vi "Controller Open Synchronization Objects.vi"(8 "error in (no error)":errorcluster, 11 "FOFB Configuration":T5={"FOFB Parameters"={"Network"={"FOFB Controller IP"="", "LNLS Control Network IP"="", "LNLS Control Network Power Supplies TCP Port"=0, "LNLS Control Network FOFB Configuration TCP Port"=0, "Data Server TCP Port"=0, "Monitoring Data TCP Port"=0, "Configuration GUI TCP Port"=0, "TCP Listening Timeout"=0}, "Fast Acquisition"={"Acquisition Period"=0, "Data Buffer Size"=0, "Monitoring Period"=0}, "Response Matrix Measurement"={"Step Amplitude"=0.0, "Time Between Steps"=0, "Step Duration"=0, "Number of Averages"=0}, "Correction Algorithm"={"Correction Period"=0, "Reference Orbit Path"=path "", "Response Matrix Path"=path "", "Correction Matrix Path"=path "", "Horizontal Correction Factor"=0.0, "Vertical Correction Factor"=0.0, "Beam Current FOFB Threshold"=0.0, "Decouple H-V"=FALSE, "Use Additional BPM LPF"=FALSE, "BPM LPF Cutoff"=0.0}, "Acquisition Network"=[], "Actuation Network"=[]}, "Number of Acquisition Chassis"=0, "Number of Actuation Chassis"=0, "Number of BPM Readings"=0, "BPM Reading Names"=[], "Selected BPM Readings"=[0, 1, 2, 3, 4, 5, 6, 7, 8, 9, 10, 11, 12, 13, 14, 15, 16, 17, 18, 19, 20, 21, 22, 23, 24, 25, 26, 27, 28, 29, 30, 31, 32, 33, 34, 35, 36, 37, 38, 39, 40, 41, 42, 43, 44, 45, 46, 47, 48, 49], "Number of Correctors"=0, "Corrector Names"=[], "Selected Correctors"=[0, 1, 2, 3, 4, 5, 6, 7, 8, 9, 10, 11, 12, 13, 14, 15, 16, 17, 18, 19, 20, 21, 22, 23, 24, 25, 26, 27, 28, 29, 30, 31, 32, 33, 34, 35, 36, 37, 38, 39, 40, 41, 42, 43, 44, 45, 46, 47, 48, 49], "Reference Orbit"=[], "Response Matrix"=[], "Correction Matrix"=[], "Acquisition Chassis Names"=[], "Actuation Chassis Names"=[], "Acquisition Variables"=[], "Actuation Variables"=[], "PS Matrix Mapping"=[], "Inverse PS Matrix Mapping"=[], "Response Matrix Beam Energy (MeV)"=0.0, "PID Parameters"=[], "BPM Planes"=[], "Corrector Planes"=[], "RMM Step Factor"=[]}) -> (0 "error out":errorcluster, 3 "Sync Objects":T1)   [LabVIEW 2011, in "Controller VIs.lvlib"]
uses:
  Controller VIs.lvlib
  Types Definitions/Type FOFB Configuration.ctl
  Types Definitions/Type FOFB Parameters.ctl
  Types Definitions/Type Network Configuration.ctl
  Types Definitions/Type FA Configuration.ctl
  Types Definitions/Type Response Matrix Measurement Configuration.ctl
  Types Definitions/Type Correction Algorithm Configuration.ctl
  Types Definitions/Type Acquisition Network Configuration.ctl
  Types Definitions/Type Actuation Network Configuration.ctl
  Types Definitions/Type PID Parameters.ctl
  Types Definitions/Type Synchronization Objects.ctl
  Types Definitions/Type Blocking Synchronization Objects.ctl
  Types Definitions/Type FA Request Parameters.ctl
  Types Definitions/Type BPM and PS select cluster.ctl
  Types Definitions/Type FA File Parameters.ctl
  Types Definitions/Type Monitoring Data.ctl
  Types Definitions/Type Diagnostics Data.ctl
  Types Definitions/Type CPU Loads Array.ctl
  Types Definitions/Type CPU Loads.ctl
  Types Definitions/Type Non-blocking Synchronization Objects.ctl
  Types Definitions/Type FOFB Variables.ctl
  Types Definitions/Type Actuation State.ctl
  Type Definitions.lvlib
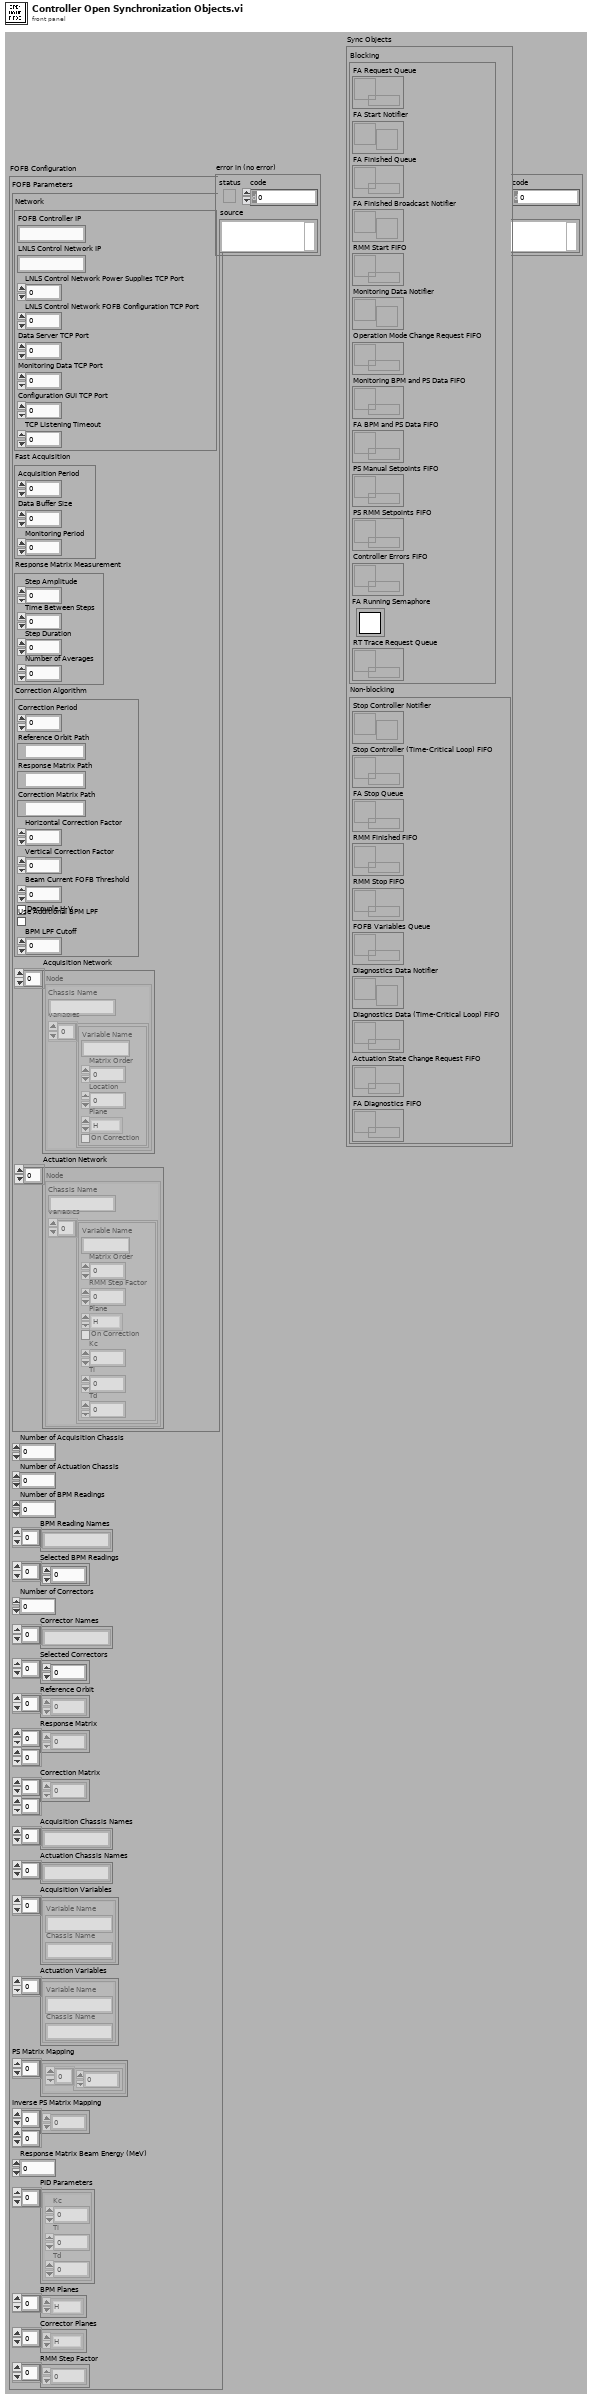
[diagram p1: front panel]
types:
  T1 = typedef "Type Definitions.lvlib/Type Synchronization Objects.ctl" = cluster{"Blocking":T2, "Non-blocking":T4}
  T2 = typedef "Type Definitions.lvlib/Type Blocking Synchronization Objects.ctl" = cluster{"FA Request Queue":refnum<queue>, "FA Start Notifier":refnum<notifier>, "FA Finished Queue":refnum<queue>, "FA Finished Broadcast Notifier":refnum<notifier>, "RMM Start FIFO":refnum<k33>, "Monitoring Data Notifier":refnum<notifier>, "Operation Mode Change Request FIFO":refnum<k33>, "Monitoring BPM and PS Data FIFO":refnum<k33>, "FA BPM and PS Data FIFO":refnum<k33>, "PS Manual Setpoints FIFO":refnum<k33>, "PS RMM Setpoints FIFO":refnum<k33>, "Controller Errors FIFO":refnum<k33>, "FA Running Semaphore":T3, "RT Trace Request Queue":refnum<queue>}
  T3 = typedef "Semaphore RefNum" = refnum<k1>
  T4 = typedef "Type Definitions.lvlib/Type Non-blocking Synchronization Objects.ctl" = cluster{"Stop Controller Notifier":refnum<notifier>, "Stop Controller (Time-Critical Loop) FIFO":refnum<k33>, "FA Stop Queue":refnum<queue>, "RMM Finished FIFO":refnum<k33>, "RMM Stop FIFO":refnum<k33>, "FOFB Variables Queue":refnum<queue>, "Diagnostics Data Notifier":refnum<notifier>, "Diagnostics Data (Time-Critical Loop) FIFO":refnum<k33>, "Actuation State Change Request FIFO":refnum<k33>, "FA Diagnostics FIFO":refnum<k33>}
  T5 = typedef "Type Definitions.lvlib/Type FOFB Configuration.ctl" = cluster{"FOFB Parameters":T6, "Number of Acquisition Chassis":i32, "Number of Actuation Chassis":i32, "Number of BPM Readings":i32, "BPM Reading Names":string[], "Selected BPM Readings":u32[], "Number of Correctors":i32, "Corrector Names":string[], "Selected Correctors":u32[], "Reference Orbit":dbl[], "Response Matrix":dbl[][], "Correction Matrix":dbl[][], "Acquisition Chassis Names":string[], "Actuation Chassis Names":string[], "Acquisition Variables":cluster{"Variable Name":string, "Chassis Name":string}[], "Actuation Variables":cluster{"Variable Name":string, "Chassis Name":string}[], "PS Matrix Mapping":cluster{u32[]}[], "Inverse PS Matrix Mapping":u32[][], "Response Matrix Beam Energy (MeV)":dbl, "PID Parameters":T13[], "BPM Planes":enum8{"H", "V"}[], "Corrector Planes":enum8{"H", "V"}[], "RMM Step Factor":dbl[]}
  T6 = typedef "Type Definitions.lvlib/Type FOFB Parameters.ctl" = cluster{"Network":T7, "Fast Acquisition":T8, "Response Matrix Measurement":T9, "Correction Algorithm":T10, "Acquisition Network":T11, "Actuation Network":T12}
  T7 = typedef "Type Definitions.lvlib/Type Network Configuration.ctl" = cluster{"FOFB Controller IP":string, "LNLS Control Network IP":string, "LNLS Control Network Power Supplies TCP Port":u16, "LNLS Control Network FOFB Configuration TCP Port":u16, "Data Server TCP Port":u16, "Monitoring Data TCP Port":u16, "Configuration GUI TCP Port":u16, "TCP Listening Timeout":i32}
  T8 = typedef "Type Definitions.lvlib/Type FA Configuration.ctl" = cluster{"Acquisition Period":u32, "Data Buffer Size":u32, "Monitoring Period":u32}
  T9 = typedef "Type Definitions.lvlib/Type Response Matrix Measurement Configuration.ctl" = cluster{"Step Amplitude":dbl, "Time Between Steps":u32, "Step Duration":u32, "Number of Averages":u32}
  T10 = typedef "Type Definitions.lvlib/Type Correction Algorithm Configuration.ctl" = cluster{"Correction Period":u32, "Reference Orbit Path":path, "Response Matrix Path":path, "Correction Matrix Path":path, "Horizontal Correction Factor":dbl, "Vertical Correction Factor":dbl, "Beam Current FOFB Threshold":dbl, "Decouple H-V":bool, "Use Additional BPM LPF":bool, "BPM LPF Cutoff":dbl}
  T11 = typedef "Type Definitions.lvlib/Type Acquisition Network Configuration.ctl" = cluster{"Chassis Name":string, "Variables":cluster{"Variable Name":string, "Matrix Order":u32, "Location":dbl, "Plane":enum8{"H", "V"}, "On Correction":bool}[]}[]
  T12 = typedef "Type Definitions.lvlib/Type Actuation Network Configuration.ctl" = cluster{"Chassis Name":string, "Variables":cluster{"Variable Name":string, "Matrix Order":u32, "RMM Step Factor":dbl, "Plane":enum8{"H", "V"}, "On Correction":bool, "Kc":dbl, "Ti":dbl, "Td":dbl}[]}[]
  T13 = typedef "Type Definitions.lvlib/Type PID Parameters.ctl" = cluster{"Kc":fxp<+/-,16,8>, "Ti":fxp<+/-,16,8>, "Td":fxp<+/-,16,8>}
  T14 = typedef "Type Definitions.lvlib/Type FOFB Variables.ctl" = cluster{"Correction Period":u32, "Reference Orbit":dbl[], "Response Matrix":dbl[][], "Correction Matrix":dbl[][], "Decouple H-V":bool, "Horizontal Correction Factor":dbl, "Vertical Correction Factor":dbl, "Selected BPM Readings":u32[], "Selected Correctors":u32[], "BPM Planes":enum8{"H", "V"}[], "Corrector Planes":enum8{"H", "V"}[], "Beam Current FOFB Threshold":dbl, "Response Matrix Beam Energy (MeV)":dbl}
  T15 = typedef "Type Definitions.lvlib/Type FA File Parameters.ctl" = cluster{"FA Parameters":T16, "File Reference":refnum<file>}
  T16 = typedef "Type Definitions.lvlib/Type FA Request Parameters.ctl" = cluster{"Number of Samples":u32, "BPM and PS Selection":T17, "Filename":string}
  T17 = typedef "Type Definitions.lvlib/Type BPM and PS select cluster.ctl" = cluster{"BPM index array":u32[], "PS index array ":u32[]}
  T18 = cluster{"read mode":enum16{"polling", "blocking"}, "write mode":enum16{"polling", "blocking"}}
  T19 = typedef "Type Definitions.lvlib/Type Diagnostics Data.ctl" = cluster{"Time-Critical Loop Missed Iterations":u32, "Time-Critical Loop Execution Time (usec)":u32, "FA Buffer Usage":u32, "Available Memory (bytes)":u32, "CPU Loads Array":T20}
  T20 = typedef "Type Definitions.lvlib/Type CPU Loads Array.ctl" = T21[]
  T21 = typedef "Type Definitions.lvlib/Type CPU Loads.ctl" = cluster{"Total (%)":dbl, "Time Critical (%)":dbl, "Timed Structures (%)":dbl, "High (%)":dbl, "Above Normal (%)":dbl, "Normal (%)":dbl, "Background (%)":dbl, "Idle (%)":dbl, "ISR (%)":dbl}
  T22 = typedef "Type Definitions.lvlib/Type Monitoring Data.ctl" = cluster{"Timestamp":timestamp, "BPM Readings":dbl[], "PS Readings":dbl[], "PS FOFB Setpoints":dbl[], "PS Status per Rack":u8[], "PS ON-OFF per Rack":u8[], "Operation Mode":enum16{"Idle Mode", "Error Mode", "Manual Mode", "FOFB Mode", "RMM Mode"}, "Diagnostics Data":T19, "Controller Status Table":i32[]}
  T23 = enum16{"Idle Mode", "Error Mode", "Manual Mode", "FOFB Mode", "RMM Mode"}
  T24 = typedef "Type Definitions.lvlib/Type Actuation State.ctl" = enum16{"Only reading", "Manual", "FOFB Initialization", "FOFB", "FOFB Stopping", "RMM Initialization", "RMM", "RMM Stopping"}
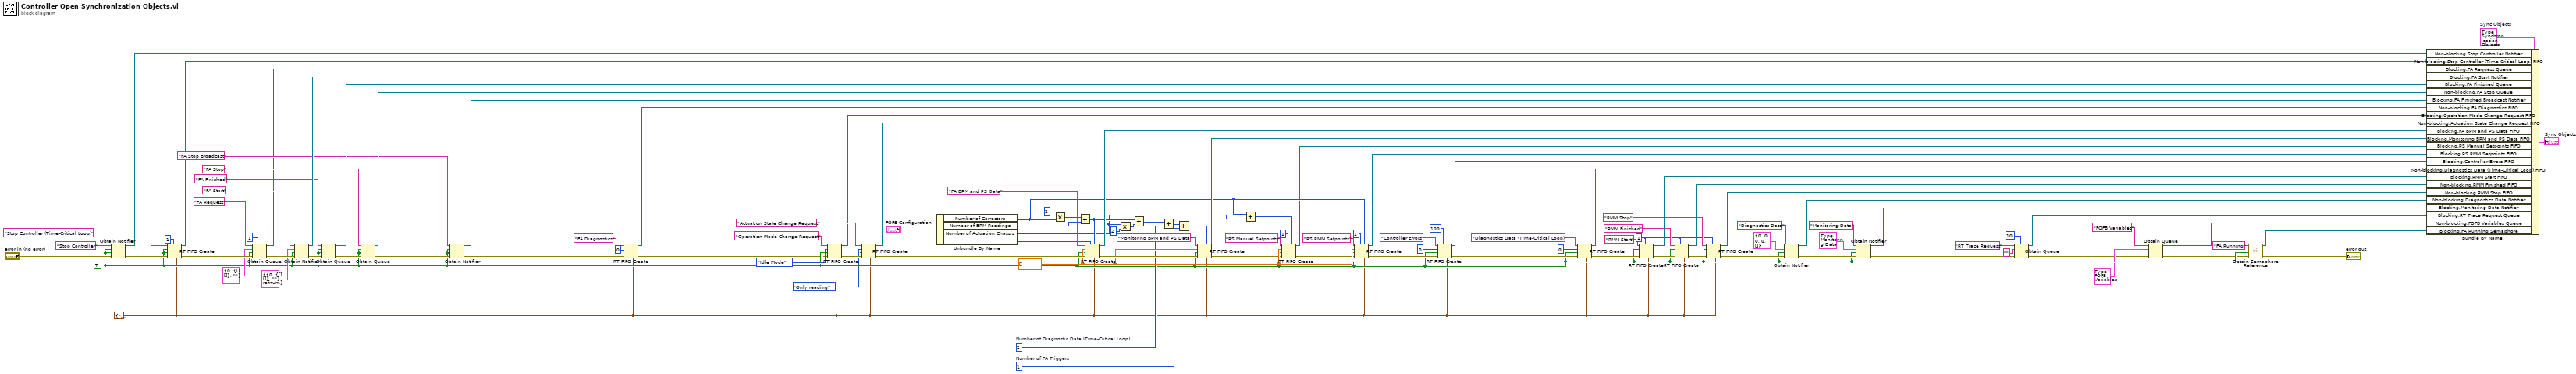
[diagram p0: block diagram]
diagram:
  w7 = 1  # Number of FA Triggers
  w30 = 2  # Number of Diagnostic Data (Time-Critical Loop)
  w11 = T18 {"read mode"=enum."blocking", "write mode"=enum."blocking"} ("r/w modes (polling,polling)")
  w58 = u32 1 ("size (10)")
  w104 = T1 {"Blocking"={"FA Request Queue"=refnum, "FA Start Notifier"=refnum, "FA Finished Queue"=refnum, "FA Finished Broadcast Notifier"=refnum, "RMM Start FIFO"=refnum, "Monitoring Data Notifier"=refnum, "Operation Mode Change Request FIFO"=refnum, "Monitoring BPM and PS Data FIFO"=refnum, "FA BPM and PS Data FIFO"=refnum, "PS Manual Setpoints FIFO"=refnum, "PS RMM Setpoints FIFO"=refnum, "Controller Errors FIFO"=refnum, "FA Running Semaphore"=refnum, "RT Trace Request Queue"=refnum}, "Non-blocking"={"Stop Controller Notifier"=refnum, "Stop Controller (Time-Critical Loop) FIFO"=refnum, "FA Stop Queue"=refnum, "RMM Finished FIFO"=refnum, "RMM Stop FIFO"=refnum, "FOFB Variables Queue"=refnum, "Diagnostics Data Notifier"=refnum, "Diagnostics Data (Time-Critical Loop) FIFO"=refnum, "Actuation State Change Request FIFO"=refnum, "FA Diagnostics FIFO"=refnum}}  # Sync Objects
  w22 = TRUE
  w46 = dbl[] [] ("BPM Readings")
  n1 = Obtain Notifier(name (unnamed)="Stop Controller", notification data type=w22, create if not found? (T)=w22, error in (no error)="error in (no error)") -> (notifier out=w105:refnum<notifier>, error out=w56:errorcluster)  [unwired: 1 out]
  n2 = RT FIFO Create(0:"Stop Controller (Time-Critical Loop)" ("name (unnamed)"), 1:w22, 2:w22, 3:w56, 4:u32 1 ("size (10)"), 7:w11) -> (8:w52:refnum<k33>, 11:w55:errorcluster)  [unwired: 2 in, 1 out]
  n3 = Obtain Queue(max queue size (-1, unlimited)=1, name (unnamed)="FA Request", element data type=T16 {"Number of Samples"=0, "BPM and PS Selection"={"BPM index array"=[], "PS index array "=[]}, "Filename"=""} ("Acquisition Period"), create if not found? (T)=w22, error in (no error)=w55) -> (queue out=w16:refnum<queue>, error out=w97:errorcluster)  [unwired: 1 out]
  n4 = Obtain Notifier(name (unnamed)="FA Start", notification data type=T15 {"FA Parameters"={"Number of Samples"=0, "BPM and PS Selection"={"BPM index array"=[], "PS index array "=[]}, "Filename"=""}, "File Reference"=refnum} ("File Parameters"), create if not found? (T)=w22, error in (no error)=w97) -> (notifier out=w106:refnum<notifier>, error out=w109:errorcluster)  [unwired: 1 out]
  n5 = Obtain Queue(name (unnamed)="FA Finished", element data type=w22, create if not found? (T)=w22, error in (no error)=w109) -> (queue out=w29:refnum<queue>, error out=w87:errorcluster)  [unwired: 1 in, 1 out]
  n6 = Obtain Queue(name (unnamed)="FA Stop", element data type=w22, create if not found? (T)=w22, error in (no error)=w87) -> (queue out=w86:refnum<queue>, error out=w25:errorcluster)  [unwired: 1 in, 1 out]
  n7 = Obtain Notifier(name (unnamed)="FA Stop Broadcast", notification data type=w22, create if not found? (T)=w22, error in (no error)=w25) -> (notifier out=w24:refnum<notifier>, error out=w13:errorcluster)  [unwired: 1 out]
  n8 = RT FIFO Create(0:"FA Diagnostics" ("name (unnamed)"), 1:0 ("# elements"), 3:w13, 7:w11) -> (8:w10:refnum<k33>, 11:w12:errorcluster)  [unwired: 4 in, 1 out]
  n9 = RT FIFO Create(0:"Operation Mode Change Request" ("name (unnamed)"), 1:T23."Idle Mode" ("Operation Mode"), 2:w22, 3:w12, 7:w11) -> (8:w81:refnum<k33>, 11:w92:errorcluster)  [unwired: 3 in, 1 out]
  n10 = RT FIFO Create(0:"Actuation State Change Request" ("name (unnamed)"), 1:Type_Actuation_State."Only reading" ("Actuation State"), 2:w22, 3:w92, 7:w11) -> (8:w80:refnum<k33>, 11:w74:errorcluster)  [unwired: 3 in, 1 out]
  n11 = Unbundle By Name("FOFB Configuration") -> ("Number of Correctors"=w43:i32, "Number of BPM Readings"=w72:i32, "Number of Actuation Chassis"=w38:i32, "FOFB Parameters.Fast Acquisition.Data Buffer Size"=w71:u32)
  n12 = Multiply(x=2 ("y"), y=w43) -> (x*y=w73:i32)
  n13 = Add(x=w73, y=w72) -> (x+y=w61:i32)
  n14 = RT FIFO Create(0:"FA BPM and PS Data" ("name (unnamed)"), 1:w46, 2:w22, 3:w74, 4:w71, 6:w61, 7:w11) -> (8:w110:refnum<k33>, 11:w77:errorcluster)  [unwired: 1 in, 1 out]
  n15 = Multiply(x=w38, y=2) -> (x*y=w39:i32)
  n16 = Add(x=w61, y=w39) -> (x+y=w31:i32)
  n17 = Add(x=w31, y=w30) -> (x+y=w9:i32)
  n18 = Add(x=w9, y=w7) -> (x+y=w8:i32)
  n19 = RT FIFO Create(0:"Monitoring BPM and PS Data" ("name (unnamed)"), 1:w46, 2:w22, 3:w77, 6:w8, 7:w11) -> (8:w76:refnum<k33>, 11:w45:errorcluster)  [unwired: 2 in, 1 out]
  n20 = Add(x=w43, y=w38) -> (x+y=w42:i32)
  n21 = RT FIFO Create(0:"PS Manual Setpoints" ("name (unnamed)"), 1:w46, 2:w22, 3:w45, 4:u32 1 ("size (10)"), 6:w42) -> (8:w41:refnum<k33>, 11:w44:errorcluster)  [unwired: 2 in, 1 out]
  n22 = RT FIFO Create(0:"PS RMM Setpoints" ("name (unnamed)"), 1:w46, 2:w22, 3:w44, 4:u32 1 ("size (10)"), 6:w43, 7:w11) -> (8:w40:refnum<k33>, 11:w51:errorcluster)  [unwired: 1 in, 1 out]
  n23 = RT FIFO Create(0:"Controller Errors" ("name (unnamed)"), 1:0 ("elements in array (1)"), 2:w22, 3:w51, 4:u32 100 ("elements in array (1)"), 7:w11) -> (8:w67:refnum<k33>, 11:w34:errorcluster)  [unwired: 2 in, 1 out]
  n24 = RT FIFO Create(0:"Diagnostics Data (Time-Critical Loop)" ("name (unnamed)"), 1:u32 0 ("elements in array (1)"), 2:w22, 3:w34, 7:w11) -> (8:w32:refnum<k33>, 11:w33:errorcluster)  [unwired: 3 in, 1 out]
  n25 = RT FIFO Create(0:"RMM Start" ("name (unnamed)"), 1:w22, 3:w33, 4:w58, 7:w11) -> (8:w107:refnum<k33>, 11:w102:errorcluster)  [unwired: 3 in, 1 out]
  n26 = RT FIFO Create(0:"RMM Finished" ("name (unnamed)"), 1:w22, 3:w102, 4:w58, 7:w11) -> (8:w108:refnum<k33>, 11:w90:errorcluster)  [unwired: 3 in, 1 out]
  n27 = RT FIFO Create(0:"RMM Stop" ("name (unnamed)"), 1:w22, 3:w90, 4:w58, 7:w11) -> (8:w89:refnum<k33>, 11:w64:errorcluster)  [unwired: 3 in, 1 out]
  n28 = Obtain Notifier(name (unnamed)="Diagnostics Data", notification data type=T19 {"Time-Critical Loop Missed Iterations"=0, "Time-Critical Loop Execution Time (usec)"=0, "FA Buffer Usage"=0, "Available Memory (bytes)"=0, "CPU Loads Array"=[]} ("Diagnostics Data"), create if not found? (T)=w22, error in (no error)=w64) -> (notifier out=w62:refnum<notifier>, error out=w63:errorcluster)  [unwired: 1 out]
  n29 = Obtain Notifier(name (unnamed)="Monitoring Data", notification data type=T22 {"Timestamp"=timestamp(0 s since 1904-01-01), "BPM Readings"=[], "PS Readings"=[], "PS FOFB Setpoints"=[], "PS Status per Rack"=[], "PS ON-OFF per Rack"=[], "Operation Mode"=enum."Idle Mode", "Diagnostics Data"={"Time-Critical Loop Missed Iterations"=0, "Time-Critical Loop Execution Time (usec)"=0, "FA Buffer Usage"=0, "Available Memory (bytes)"=0, "CPU Loads Array"=[]}, "Controller Status Table"=[]} ("Slow Data"), create if not found? (T)=w22, error in (no error)=w63) -> (notifier out=w83:refnum<notifier>, error out=w4:errorcluster)  [unwired: 1 out]
  n30 = Obtain Queue(max queue size (-1, unlimited)=10, name (unnamed)="RT Trace Request", element data type="" ("Host IP Address"), error in (no error)=w4) -> (queue out=w1:refnum<queue>, error out=w3:errorcluster)  [unwired: 1 in, 1 out]
  n31 = Obtain Queue(name (unnamed)="FOFB Variables", element data type=T14 {"Correction Period"=0, "Reference Orbit"=[], "Response Matrix"=[], "Correction Matrix"=[], "Decouple H-V"=FALSE, "Horizontal Correction Factor"=0.0, "Vertical Correction Factor"=0.0, "Selected BPM Readings"=[], "Selected Correctors"=[], "BPM Planes"=[], "Corrector Planes"=[], "Beam Current FOFB Threshold"=0.0, "Response Matrix Beam Energy (MeV)"=0.0} ("FOFB Variables 2"), error in (no error)=w3) -> (queue out=w17:refnum<queue>, error out=w21:errorcluster)  [unwired: 2 in, 1 out]
  n32 = call <vilib>:"Obtain Semaphore Reference.vi"("error in (no error)"=w21, "create if not found (T)"=w22, "name (unnamed)"="FA Running") -> ("error out"=→"error out":errorcluster, "semaphore"=w18:T3)  [unwired: 2 in, 1 out]
  n33 = Bundle By Name(cluster=w104, "Non-blocking.Stop Controller Notifier"=w105, "Non-blocking.Stop Controller (Time-Critical Loop) FIFO"=w52, "Blocking.FA Request Queue"=w16, "Blocking.FA Start Notifier"=w106, "Blocking.FA Finished Queue"=w29, "Non-blocking.FA Stop Queue"=w86, "Blocking.FA Finished Broadcast Notifier"=w24, "Non-blocking.FA Diagnostics FIFO"=w10, "Blocking.Operation Mode Change Request FIFO"=w81, "Non-blocking.Actuation State Change Request FIFO"=w80, "Blocking.FA BPM and PS Data FIFO"=w110, "Blocking.Monitoring BPM and PS Data FIFO"=w76, "Blocking.PS Manual Setpoints FIFO"=w41, "Blocking.PS RMM Setpoints FIFO"=w40, "Blocking.Controller Errors FIFO"=w67, "Non-blocking.Diagnostics Data (Time-Critical Loop) FIFO"=w32, "Blocking.RMM Start FIFO"=w107, "Non-blocking.RMM Finished FIFO"=w108, "Non-blocking.RMM Stop FIFO"=w89, "Non-blocking.Diagnostics Data Notifier"=w62, "Blocking.Monitoring Data Notifier"=w83, "Blocking.RT Trace Request Queue"=w1, "Non-blocking.FOFB Variables Queue"=w17, "Blocking.FA Running Semaphore"=w18) -> (→"Sync Objects":T1)
